vi "DataAcquisition.vi"(6 "stop":bool, 9 "linesPerUpdate":u16=1) -> (4 "lineIndex":u32)   [LabVIEW 2016]
uses:
  controls/FPGAVIreferenceTypeDef.ctl
  controls/Enum.ctl
  <vilib>/Utility/error.llb/Error Cluster From Error Code.vi
  <vilib>/rvi/errors/niLvFpgaAdjustHostInterfaceError.vi
  <vilib>/rvi/interface/common/niFpgaWaitOnOcc.vi
  <vilib>/rvi/interface/nirviMethod/nirviMethod.xnode
  FPGA Bitfiles/qnmController797_usbRIO_controllerFPGAmu.lvbitx
  controls/FPGAVIreferenceTypeDefScanEngine.ctl
  <vilib>/rvi/interface/nirviReadWriteControl/nirviReadWriteControl.xnode
  <vilib>/rvi/errors/niLvFpgaMergeErrorWithErrorCode.vi
  NiFpgaLv.dll
  <vilib>/FPGAPlugInAG/USB-7856R OEM/niLvFpga_ConfigureFifo_USB-7856R OEM.vi
  <vilib>/FPGAPlugInAG/USB-7856R OEM/niLvFpga_StopFifo_USB-7856R OEM.vi
panel:
  out "eltsRemaining":u32
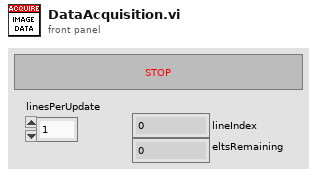
[diagram p1: front panel]
types:
  T1 = typedef "Enum.ctl" = enum16{"Init", "Read", "Write"}
  T2 = typedef "FPGAVIreferenceTypeDef.ctl" = refnum<k20>
  T3 = typedef "FPGAVIreferenceTypeDefScanEngine.ctl" = refnum<k20>
  T4 = typedef "ScanWaveform.ctl" = enum16{"Sine", "Triangle", "Rounded"}
  T5 = cluster{"slowWavePts":u16, "fastWavePts":u16, "slowWaveType":T4, "fastWaveType":T4, "slowRoundPts":u16, "fastRoundPts":u16, "singleDirectionScan":bool}
  T6 = cluster{"Width":dbl, "Height":dbl, "X Offset":dbl, "Y Offset":dbl, "Angle":dbl, "Pixels/Line":u16, "Lines":u16, "Time/Line":dbl, "Scan Rate":dbl}
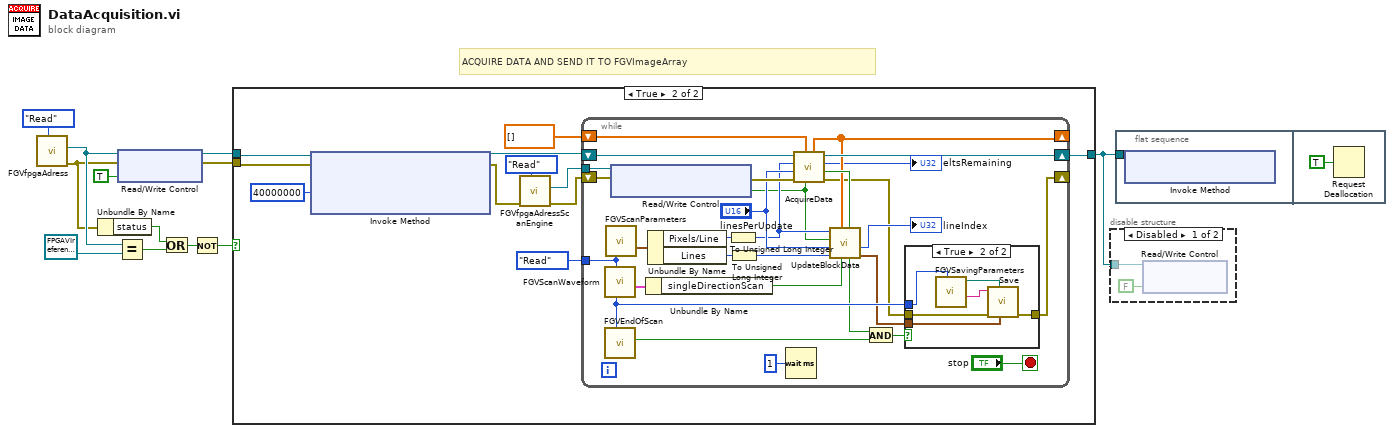
[diagram p0: block diagram]
diagram:
  # "ACQUIRE DATA AND SEND IT TO FGVImageArray"
  n1 = call "FGVfpgaAdress.vi"("Enum"=Enum."Read") -> ("error out"=w6:errorcluster, "FPGA VI Reference Out"=w7:T2)  [unwired: 5 in, 4 out]
  n2 = Unbundle By Name(w6) -> ("status"=w10:bool)
  n3 = Equal?(x=w7, y=T2 refnum ("FPGA VI Reference Out")) -> (x = y?=w9:bool)
  n4 = xnode "Read/Write Control"("FPGA VI Reference In"=w7, "error in"=w6, "hdt.o.enable"=TRUE) -> ("FPGA VI Reference Out"=w5:T2, "error out"=w4:errorcluster)
  n5 = Or(x=w10, y=w9) -> (x .or. y?=w11:bool)
  n6 = Not(x=w11) -> (.not. x?=w8:bool)
  n7 = case shown="True" w8 {
    tunnel: w5 -> [w13 w23]
    tunnel: w4 -> [_ w24]
    tunnel: [w13 w20] -> w2
    frame False {
    }
    frame True {
      n8 = xnode "Invoke Method"("FPGA VI Reference In"=w23, "error in"=w24, "Requested Depth"=u32 40000000) -> ("FPGA VI Reference Out"=w21:T2, "error out"=w14:errorcluster)  [unwired: 1 out]
      n9 = call "FGVfpgaAdressScanEngine.vi"("Enum"=Enum."Read", "error in"=w14) -> ("error out"=w15:errorcluster, "FPGA.SEout"=w17:T3)  [unwired: 5 in, 3 out]
      n10 = while {
        tunnel: Enum."Read" ("Enum") -> [w51]
        shift-right: [w44] -> w20
        shift-left: w21 -> [w45]
        tunnel: w17 -> [w35]
        shift-right: [w33] -> _
        shift-left: sgl[] [] ("DataIn") -> [w34]
        shift-right: [w25] -> _
        shift-left: w15 -> [w31]
        stop <- "stop" stop-if-true
        n11 = call "FGVScanWaveform.vi"("Enum"=w51) -> ("scanWaveFormCtl Out"=w47:T5)  [unwired: 9 in, 1 out]
        n12 = call "FGVEndOfScan.vi"("Enum"=w51) -> ("autoSaveOut"=w43:bool)  [unwired: 9 in, 1 out]
        n13 = call "FGVScanParameters.vi"("Enum"=w51) -> ("Scan Parameters Out"=w48:T6)  [unwired: 9 in, 1 out]
        n14 = xnode "Read/Write Control"("FPGA VI Reference In"=w35, "error in"=w31) -> ("error out"=w52:errorcluster, "se.p.modes.se.p.enable"=w32:bool)  [unwired: 1 out]
        n15 = Unbundle By Name(w47) -> ("singleDirectionScan"=w46:bool)
        n16 = Unbundle By Name(w48) -> ("Pixels/Line"=w37:u16, "Lines"=w50:u16)
        n17 = To Unsigned Long Integer(number=w37) -> (unsigned 32bit integer=w36:u32)
        n18 = To Unsigned Long Integer(number=w50) -> (unsigned 32bit integer=w40:u32)
        n19 = Wait (ms)(milliseconds to wait=u32 1) -> ()  [unwired: 1 out]
        n20 = call "AcquireData.vi"("ScanEnable"=w32, "DataIn"=w34, "error in"=w52, "linesPerUpdate"="linesPerUpdate", "Pixels/Line"=w36, "FPGA VI Reference In"=w45) -> ("error out"=w26:errorcluster, "BlockUpdate?"=w38:bool, "Elements Remaining"=→"eltsRemaining":u32, "FPGA VI Reference Out"=w44:T2, "DataOut"=w33:sgl[])  [unwired: 1 in]
        n21 = call "UpdateBlockData.vi"("BlockUpdate"=w38, "singleDirectionScan"=w46, "Data"=w33, "Lines"=w40, "linesPerUpdate"="linesPerUpdate", "ScanEnable?"=w32, "Pixels/Line"=w36) -> ("current time"=w29:timestamp, "LineIndex"=→"lineIndex":u32, "EndOfScan?"=w41:bool)  [unwired: 2 in]
        n22 = And(x=w41, y=w43) -> (x .and. y?=w42:bool)
        n23 = case shown="True" w42 {
          tunnel: w29 -> [_ w59]
          tunnel: w51 -> [_ w56]
          tunnel: w26 -> [w53 w55]
          tunnel: [w53 w54] -> w25
          frame False {
          }
          frame True {
            n24 = call "FGVSavingParameters.vi"("Enum"=w56) -> ("filenameOut"=w58:string, "pathOut"=w57:path)  [unwired: 7 in, 2 out]
            n25 = call "Save.vi"("current time"=w59, "base path"=w57, "error in"=w55, "Filename"=w58) -> ("error out"=w54:errorcluster)  [unwired: 6 in, 1 out]
          }
        }
      }
    }
  }
  n26 = disable-structure shown="Disabled" {
    disable-tunnel: w2 -> [w61 _]
    frame Disabled {
      n27 = xnode "Read/Write Control"("FPGA VI Reference In"=w61, "hdt.o.enable"=FALSE) -> ()  [unwired: 1 in, 2 out]
    }
    frame Enabled {
    }
  }
  n28 = flat-sequence {
    tunnel: w2 -> [w62]
    frame #0 {
      n29 = xnode "Invoke Method"("FPGA VI Reference In"=w62) -> ()  [unwired: 1 in, 2 out]
    }
    frame #1 {
      n30 = Request Deallocation(TRUE ("flag")) -> ()
    }
  }
